vi "ReadMessage.vi"(6 "timeout in ms (-1)":i32=-1, 8 "error in":errorcluster, 11 "message ref in":refnum<class "CLM_PriorityLocalMessage.lvclass">) -> (0 "error out":errorcluster, 1 "data":variant, 2 "name":string, 3 "message ref out":refnum<class "CLM_PriorityLocalMessage.lvclass">, 4 "timed out?":bool, 5 "priority":i32, 7 "attributes":variant)   [LabVIEW 2013, in "CLM_PriorityLocalMessage.lvclass"]
uses:
  CLM_PriorityLocalMessage.lvclass
  CLM_PriorityLocalMessage.lvclass/CLM_PriorityLocalMessage.ctl
  LocalMessage_Queue/CLM_LocalMessage_Queue.lvclass/CLM_LocalMessage_Queue.ctl
  LocalMessage_Queue/ReadQueueMessage_Cluster.vi
  BufferIndexToPriority.vi
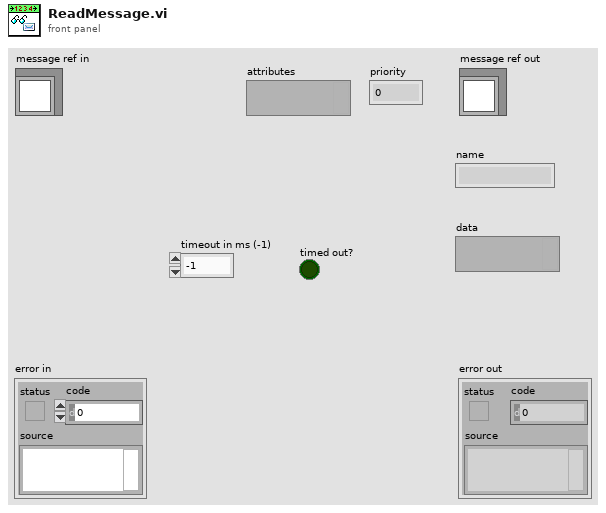
[diagram p1: front panel]
types:
  T1 = typedef "CLM_LocalMessage.lvclass/Message.ctl" = cluster{"name":string, "data":variant, "attributes":variant, "urgent":bool}
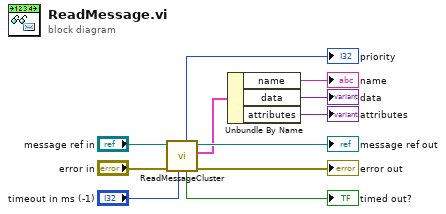
[diagram p0: block diagram]
diagram:
  n1 = call "ReadMessageCluster.vi"("timeout in ms (-1)"="timeout in ms (-1)", "error in"="error in", "queues in"="message ref in") -> ("error out"=→"error out":errorcluster, "message"=w6:T1, "queues out"=→"message ref out":refnum<class "CLM_PriorityLocalMessage.lvclass">, "timed out?"=→"timed out?":bool, "priority"=→"priority":i32)  [unwired: 4 in]
  n2 = Unbundle By Name(w6) -> ("name"=→"name":string, "data"=→"data":variant, "attributes"=→"attributes":variant)
